vi "CalcStereoDist - Copy.vi"(1 "Image Height":i32, 2 "Image Width":i32, 3 "BlobData":T1(array[cluster])) -> (0 "Distance":cluster{"Z":dbl, "Zft":dbl, "Score":dbl}[](array[cluster]))   [LabVIEW 2011]
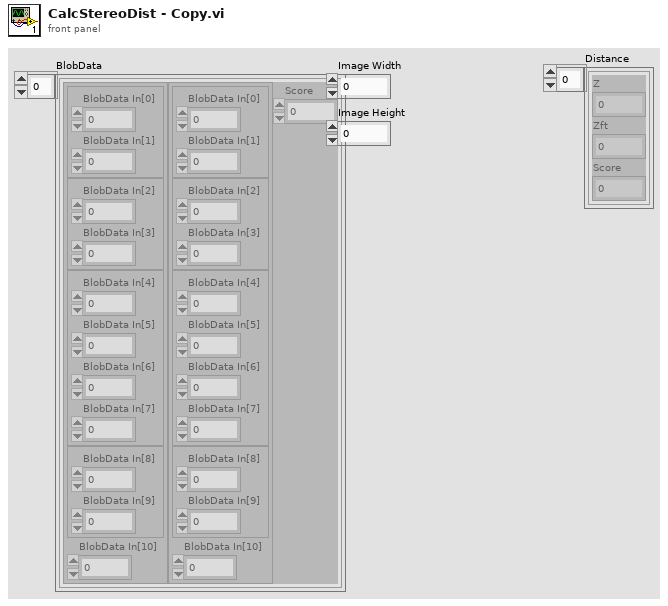
[diagram p1: front panel]
types:
  T1 = cluster{cluster{cluster{"BlobData In[0]":dbl, "BlobData In[1]":dbl}, cluster{"BlobData In[2]":dbl, "BlobData In[3]":dbl}, cluster{"BlobData In[4]":dbl, "BlobData In[5]":dbl, "BlobData In[6]":dbl, "BlobData In[7]":dbl}, cluster{"BlobData In[8]":dbl, "BlobData In[9]":dbl}, "BlobData In[10]":dbl}, cluster{cluster{"BlobData In[0]":dbl, "BlobData In[1]":dbl}, cluster{"BlobData In[2]":dbl, "BlobData In[3]":dbl}, cluster{"BlobData In[4]":dbl, "BlobData In[5]":dbl, "BlobData In[6]":dbl, "BlobData In[7]":dbl}, cluster{"BlobData In[8]":dbl, "BlobData In[9]":dbl}, "BlobData In[10]":dbl}, "Score":dbl}[]
  T2 = cluster{cluster{"BlobData In[0]":dbl, "BlobData In[1]":dbl}, cluster{"BlobData In[2]":dbl, "BlobData In[3]":dbl}, cluster{"BlobData In[4]":dbl, "BlobData In[5]":dbl, "BlobData In[6]":dbl, "BlobData In[7]":dbl}, cluster{"BlobData In[8]":dbl, "BlobData In[9]":dbl}, "BlobData In[10]":dbl}
  T3 = cluster{"BlobData In[0]":dbl, "BlobData In[1]":dbl}
  T4 = cluster{"XYZ":cluster{"X":dbl, "Y":dbl, "Z":dbl}, "XYZ (ft)":cluster{"X":dbl, "Y":dbl, "Z":dbl}, "Score":dbl}
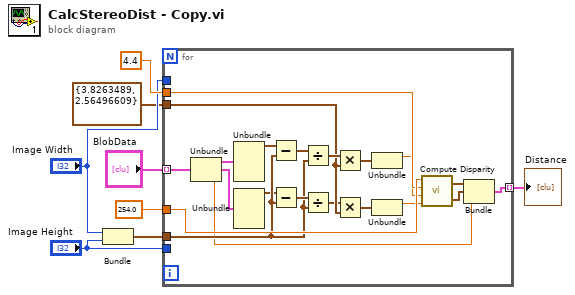
[diagram p0: block diagram]
diagram:
  n1 = Bundle("Image Width"="Image Width", "Image Height"="Image Height") -> (w3:cluster{"Image Width":i32, "Image Height":i32})  [unwired: 1 in]
  n2 = for {
    tunnel: "BlobData" -> [w10] mode=indexing
    tunnel: 254.0 ("b") -> [w29]
    tunnel: 4.4 ("f") -> [w28]
    tunnel: "Image Width" -> [_]
    tunnel: "Image Height" -> [_]
    tunnel: w3 -> [w22]
    tunnel: cluster{dbl, dbl} {3.8263489, 2.56496609} -> [w19]
    tunnel: [w12] -> w1 mode=indexing
    n3 = Unbundle(w10) -> (w27:T2, w26:T2, "Score"=w9:dbl)
    n4 = Unbundle(w27) -> (w24:T3)  [unwired: 4 out]
    n5 = Unbundle(w26) -> (w21:T3)  [unwired: 4 out]
    n6 = Subtract(x=w24, y=w22) -> (x-y=w25:cluster{dbl, dbl})
    n7 = Subtract(x=w21, y=w22) -> (x-y=w23:cluster{dbl, dbl})
    n8 = Divide(x=w25, y=w22) -> (x/y=w20:cluster{dbl, dbl})
    n9 = Divide(x=w23, y=w22) -> (x/y=w18:cluster{dbl, dbl})
    n10 = Multiply(x=w20, y=w19) -> (x*y=w17:cluster{dbl, dbl})
    n11 = Multiply(x=w18, y=w19) -> (x*y=w16:cluster{dbl, dbl})
    n12 = Unbundle(w17) -> (w15:dbl)  [unwired: 1 out]
    n13 = Unbundle(w16) -> (w14:dbl)  [unwired: 1 out]
    n14 = call "Compute Disparity.vi"("t"=w14, "r"=w15, "f"=w28, "b"=w29) -> ("XYZ (ft)"=w11:cluster{"X":dbl, "Y":dbl, "Z":dbl}, "XYZ"=w13:cluster{"X":dbl, "Y":dbl, "Z":dbl})
    n15 = Bundle("XYZ"=w13, "XYZ (ft)"=w11, "Score"=w9) -> (w12:T4)  [unwired: 1 in]
  }
  "Distance" <- w1
